vi "Test Process Reentrancy.vi"(8 "error in (no error)":errorcluster, 11 "Process Test in":refnum<class "Process Dev Test.lvclass">) -> (0 "error out":errorcluster, 3 "Process Test out":refnum<class "Process Dev Test.lvclass">)   [LabVIEW 2020, in "Process Dev Test.lvclass"]
uses:
  Process Dev Test.lvclass
  C:/Git/astemes-triarc-framework/source/Framework Test/Base Class Test/Base Test.lvclass
  C:/Program Files (x86)/National Instruments/LabVIEW 2020/vi.lib/Astemes/LUnit/Test Case.lvclass
  source/Framework Test Suite/Base Class Test/Base Test.lvclass/Base Test.ctl
  <vilib>/Astemes/LUnit/Test Case.lvclass/Test Case.ctl
  <vilib>/Astemes/LUnit/LUnit Assertion Result.lvclass/LUnit Assertion Result.ctl
  <vilib>/Astemes/LUnit/LUnit Test Case Result.lvclass/LUnit Test Case Result.ctl
  <vilib>/Astemes/LUnit/LUnit Method Result.lvclass/LUnit Method Result.ctl
  <vilib>/Astemes/LUnit/Palette/Fail.vi
  <vilib>/Astemes/LUnit/Palette/Pass.vi
  <vilib>/Astemes/LUnit/Set Assertion Type.vi
  <vilib>/Astemes/LUnit/Add test result.vi
  <vilib>/Astemes/LUnit/LUnit Write Passed.vi
  <vilib>/Astemes/LUnit/LUnit Write Message.vi
  <vilib>/Astemes/LUnit/LUnit Write Description.vi
  <vilib>/Astemes/LUnit/LUnit Write Assertion Type.vi
  <vilib>/Astemes/LUnit/LUnit Record Assertion Result.vi
  <vilib>/Astemes/LUnit/LUnit Aggregate Assertion Results.vi
  <vilib>/Astemes/LUnit/Assertion Result/LUnit Read Status.vi
  <vilib>/Astemes/LUnit/LUnit Read Message.vi
  <vilib>/Astemes/LUnit/LUnit Read Description.vi
  <vilib>/Astemes/LUnit/Method Result/LUnit Merge Status.vi
  <vilib>/Astemes/LUnit/LUnit Concatenate result strings.vi
  source/Framework/Base/Base.lvclass
  <vilib>/Astemes/LUnit/LUnit Assertion Result.lvclass
  Process Dev Test.lvclass/Process Dev Test.ctl
  <vilib>/Astemes/LUnit/Test Case.lvclass
  source/Framework Test Suite/Base Class Test/Base Test.lvclass
  C:/Git/astemes-triarc-framework/source/TF Test Suite/Base Class Test/Base Test.lvclass
  C:/Git/astemes-triarc-framework/test/Process Development Test/Process Test/Process Dev Test.lvclass
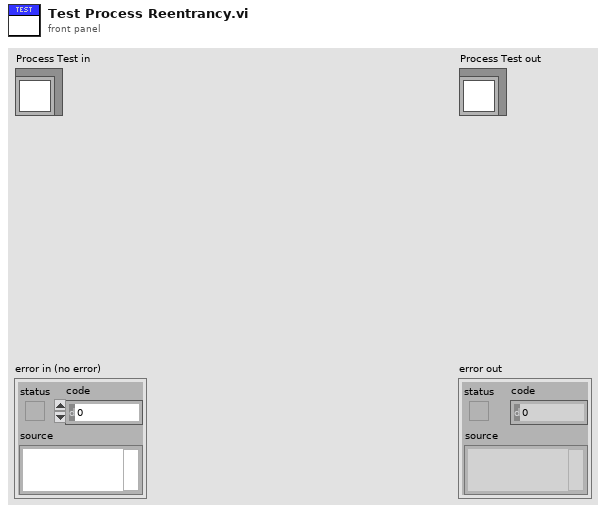
[diagram p1: front panel]
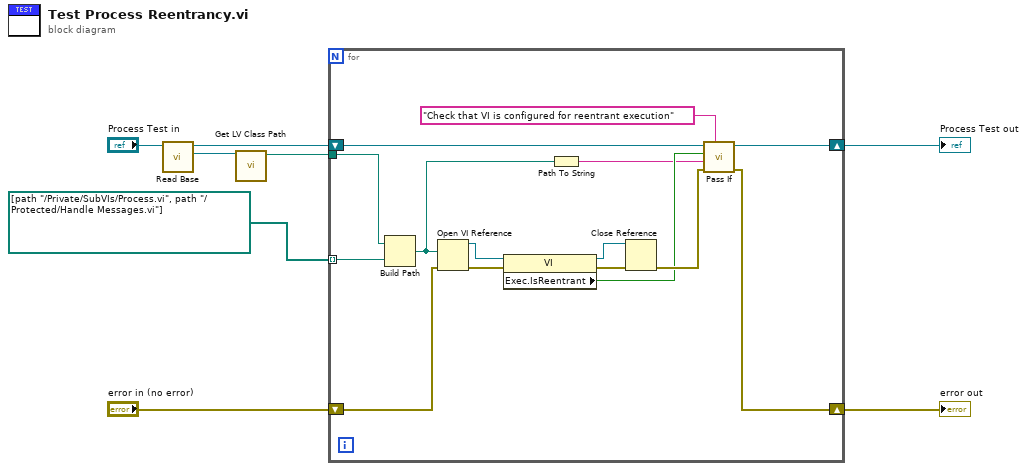
[diagram p0: block diagram]
diagram:
  n1 = call "Read Base.vi"("Base Class Test In"="Process Test in") -> ("Base.lvclass"=w3:refnum<class "Base.lvclass">, "Base Class Test Out"=w4:refnum<class "Process Dev Test.lvclass">)  [unwired: 8 in, 1 out]
  n2 = call <vilib>:"Get LV Class Path.vi"("object"=w3) -> ("class path"=w2:path)  [unwired: 9 in, 1 out]
  n3 = for {
    tunnel: w2 -> [w12]
    shift-right: [w18] -> w6
    shift-left: "error in (no error)" -> [w16]
    shift-right: [w21] -> w7
    shift-left: w4 -> [w13]
    tunnel: path[] [path "../Private/SubVIs/Process.vi", path "../Protected/Handle Messages.vi"] -> [w11] mode=indexing
    n4 = Build Path(base path=w12, name or relative path=w11) -> (appended path=w10:path)
    n5 = Open VI Reference(vi path=w10, error in (no error)=w16) -> (vi reference=w15:refnum<vi>, error out=w17:errorcluster)  [unwired: 4 in]
    n6 = property class="VI"(reference=w15, error in=w17) -> (reference out=w22:refnum<vi>, error out=w23:errorcluster, "Exec.IsReentrant"=w19:bool)
    n7 = Path To String(path=w10) -> (string=w9:string)
    n8 = Close Reference(reference=w22, error in (no error)=w23) -> (error out=w20:errorcluster)
    n9 = call <vilib>:"Pass If.vi"("Description"="Check that VI is configured for reentrant execution", "error in (no error)"=w20, "Message"=w9, "Pass?"=w19, "LUnit Test Case In"=w13) -> ("error out"=w18:errorcluster, "LUnit Test Case Out"=w21:refnum<class "Process Dev Test.lvclass">)  [unwired: 5 in]
  }
  "error out" <- w6
  "Process Test out" <- w7
